vi "曲线拆分.vi"(11 "原始曲线":cluster{dbl[], dbl[]}[](array[cluster])) -> (3 "拆分后曲线":cluster{dbl[], dbl[]}[](array[cluster]))   [LabVIEW 2020]
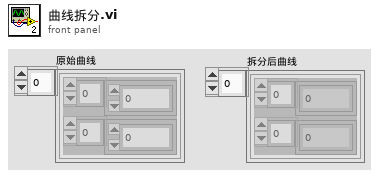
[diagram p1: front panel]
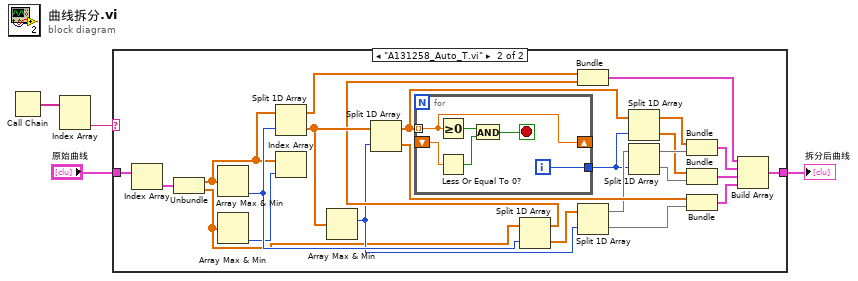
[diagram p0: block diagram]
diagram:
  n1 = Call Chain() -> (call chain=w2:string[])
  n2 = Index Array(array=w2) -> (element #2=w1:string)  [unwired: 2 in, 1 out]
  n3 = case shown="\"A131258_Auto_T.vi\"" w1 {
    tunnel: "原始曲线" -> [w5 w7]
    tunnel: [w5 w6] -> w3
    frame "假", Default {
    }
    frame "A131258_Auto_T.vi" {
      n4 = Index Array(array=w7) -> (element=w15:cluster{dbl[], dbl[]})  [unwired: 1 in]
      n5 = Unbundle(w15) -> (w9:dbl[], w10:dbl[])
      n6 = Array Max & Min(array=w9) -> (min index (indices)=w24:i32)  [unwired: 3 out]
      n7 = Array Max & Min(array=w10) -> (min index (indices)=w8:i32)  [unwired: 3 out]
      n8 = Split 1D Array(array=w9, index=w24) -> (first subarray=w28:dbl[], second subarray=w30:dbl[])
      n9 = Index Array(array=w9, index=w8) -> ()  [unwired: 1 out]
      n10 = Array Max & Min(array=w30) -> (max index (indices)=w23:i32)  [unwired: 3 out]
      n11 = Split 1D Array(array=w30, index=w23) -> (first subarray=w21:dbl[], second subarray=w26:dbl[])
      n12 = for {
        tunnel: w21 -> [w36] mode=indexing
        shift-right: [w36] -> _
        shift-left: _ -> [w35]
        tunnel: [w31] -> w20
        i -> [w31]
        stop <- w32 stop-if-true
        n13 = Greater Or Equal To 0?(x=w36) -> (x >= 0?=w34:bool)
        n14 = Less Or Equal To 0?(x=w35) -> (x <= 0?=w33:bool)
        n15 = And(x=w34, y=w33) -> (x .and. y?=w32:bool)
      }
      n16 = Split 1D Array(array=w10, index=w24) -> (first subarray=w27:dbl[], second subarray=w29:dbl[])
      n17 = Bundle(w28, w27) -> (w14:cluster{dbl[], dbl[]})  [unwired: 1 in]
      n18 = Split 1D Array(array=w29, index=w23) -> (first subarray=w22:dbl[], second subarray=w25:dbl[])
      n19 = Split 1D Array(array=w21, index=w20) -> (first subarray=w19:dbl[], second subarray=w17:dbl[])
      n20 = Split 1D Array(array=w22, index=w20) -> (first subarray=w18:dbl[], second subarray=w16:dbl[])
      n21 = Bundle(w19, w18) -> (w12:cluster{dbl[], dbl[]})  [unwired: 1 in]
      n22 = Bundle(w17, w16) -> (w11:cluster{dbl[], dbl[]})  [unwired: 1 in]
      n23 = Bundle(w26, w25) -> (w13:cluster{dbl[], dbl[]})  [unwired: 1 in]
      n24 = Build Array(w14, w12, w11, w13) -> (w6:cluster{dbl[], dbl[]}[])
    }
  }
  "拆分后曲线" <- w3
